vi "ingest.job_status.vi"(8 "error in":errorcluster, 11 "IngestJob in":refnum<class "IngestJob.lvclass">) -> (0 "error out":errorcluster, 3 "IngestJob out":refnum<class "IngestJob.lvclass">)   [LabVIEW 2020, in "IngestJob.lvclass"]
doc: "Returns the current lifecycle status of an ingest job."
uses:
  IngestJob.lvclass
  IngestJob.lvclass/IngestJob.ctl
  client.lvlib
panel:
  out "out_status out":i32
  in  "out_status":i32
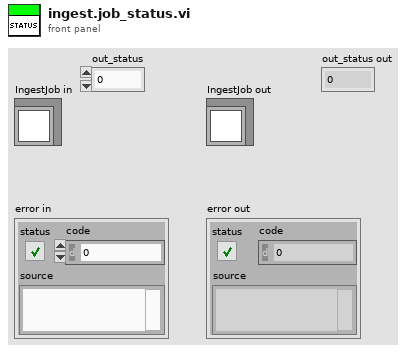
[diagram p1: front panel]
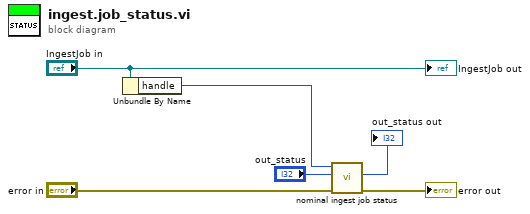
[diagram p0: block diagram]
diagram:
  n1 = Unbundle By Name("IngestJob in") -> ("handle"=w4:i32)
  n2 = call "nominal ingest job status.vi"("error in (no error)"="error in", "out_status"="out_status", "job"=w4) -> ("error out"=→"error out":errorcluster, "out_status out"=→"out_status out":i32)  [unwired: 6 in, 1 out]
  "IngestJob out" <- "IngestJob in"
